vi "UdsAttrLog.vi"(8 "This VI":refnum<vi>, 10 "Content":string, 11 "UdsHandleIn":T1) -> (3 "UdsHandleOut":T1)   [LabVIEW 2011, in "Konvolucio MUDS150628.lvlib"]
uses:
  <instrlib>/Konvolucio MUDS150628/Konvolucio MUDS150628.lvlib
  <instrlib>/Konvolucio MUDS150628/Types/UdsHandleType.ctl
  <instrlib>/Konvolucio MCAN120803/Types/MCanHandleType.ctl
  C:/Program Files/National Instruments/LabVIEW 2011/instr.lib/Konvolucio MCAN120803/Private/Konvolucio.MCAN120803.dll
  Konvolucio MCAN120803/Private/Konvolucio.MCAN120803.dll
  <instrlib>/Konvolucio MUDS150628/Private/UdsLogEvent.vi
  <instrlib>/Konvolucio MCAN120803/Konvolucio MCAN120803.lvlib
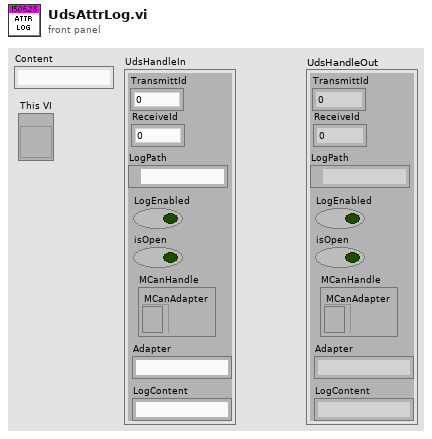
[diagram p1: front panel]
types:
  T1 = typedef "Konvolucio MUDS150628.lvlib/UdsHandleType.ctl" = cluster{"LogPath":path, "LogEnabled":bool, "isOpen":bool, "LogContent":string, "Adapter":string, "MCanHandle":T2, "TransmittId":u32, "ReceiveId":u32}
  T2 = typedef "Konvolucio MCAN120803.lvlib/MCanHandleType.ctl" = cluster{"MCanAdapter":refnum<k24>}
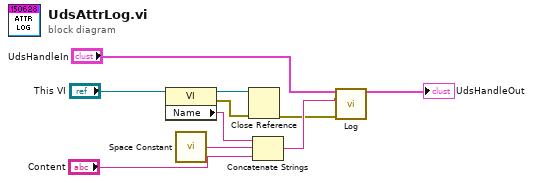
[diagram p0: block diagram]
diagram:
  n1 = property class="VI"(reference="This VI") -> (reference out=w5:refnum<vi>, error out=w6:errorcluster, "Name"=w8:string)  [unwired: 1 in]
  n2 = call <vilib>:"Space Constant.vi"() -> ("String"=w7:string)
  n3 = Close Reference(reference=w5, error in (no error)=w6) -> (error out=w2:errorcluster)
  n4 = Concatenate Strings(w8, w7, "Content") -> (w4:string)
  n5 = call-poly <instrlib>:"Log.vi"("UdsHandleIn"="UdsHandleIn", "EventMsg"=w4, "error in"=w2) -> ("UdsHandleOut"=→"UdsHandleOut":T1)  [unwired: 11 in, 1 out]
